vi "getConfig.vi"(6 "Delay between send and receive [ms]":i32=100, 8 "error in (no error)":errorcluster, 11 "Monochromator in":refnum<class "Monochromator.lvclass">) -> (0 "error out":errorcluster, 3 "Monochromator out":refnum<class "Monochromator.lvclass">)   [LabVIEW 2023, in "Monochromator.lvclass"]
uses:
  Monochromator.lvclass
  Monochromator.lvclass/Monochromator.ctl
  d9b87029-586e-44ee-a6e5-d4a5e0edce38.vi
  b59fd1e7-dcda-425c-bd6c-61aafb79e7f4.vi
  GenericDevice/GenericDevice.lvclass
  <vilib>/IlluminatedG/lv-web-crypto/lv-json/JSON/JSON.lvlib
panel:
  # "Connector Pane"
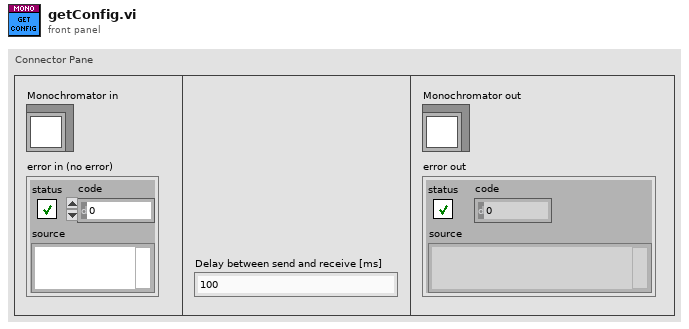
[diagram p1: front panel]
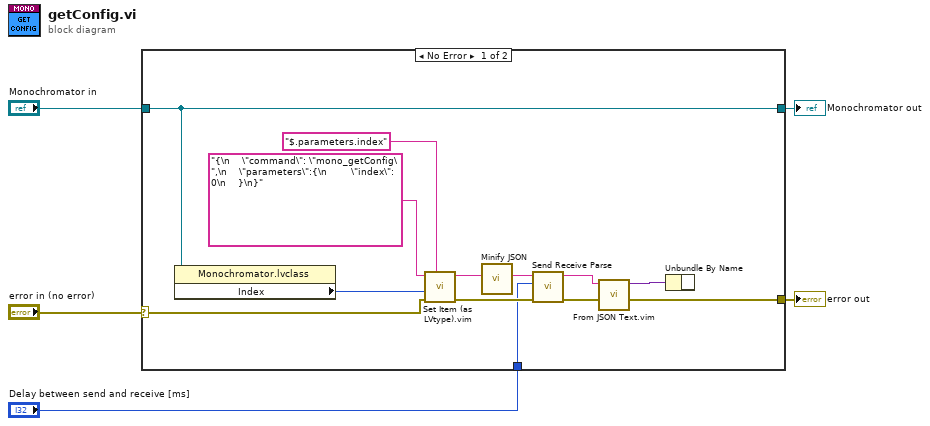
[diagram p0: block diagram]
diagram:
  n1 = case shown="No Error" "error in (no error)" {
    selector: "error in (no error)" -> [w14 w20]
    tunnel: [w13 w20] -> w4
    tunnel: [w16 w19] -> w2
    tunnel: "Monochromator in" -> [w16 w19]
    tunnel: "Delay between send and receive [ms]" -> [w6 _]
    frame No Error {
      n2 = property class="Monochromator.lvclass"(reference=w16) -> ("Index"=w15:i32)  [unwired: 1 in, 2 out]
      n3 = call "Set Item (as LVtype).vim"("$Path or Item Name"="$.parameters.index", "error in (no error)"=w14, "Anything"=w15, "JSON"="{\n    \"command\": \"mono_getConfig\",\n    \"parameters\":{\n        \"index\": 0\n    }\n}") -> ("error out"=w12:errorcluster, "<JSON>"=w9:string)  [unwired: 4 in, 1 out]
      n4 = call <vilib>:"Minify JSON.vi"("JSON String"=w9) -> ("Minified JSON"=w8:string)  [unwired: 10 in]
      n5 = call "Send Receive Parse.vi"("error in"=w12, "Delay between send and receive [ms]"=w6, "<JSON>"=w8) -> ("error out"=w10:errorcluster, "results-JSON string"=w11:string)  [unwired: 6 in, 1 out]
      n6 = call "From JSON Text.vim"("error in (no error)"=w10, "JSON"=w11) -> ("error out"=w13:errorcluster, "Data out"=w7:variant)  [unwired: 8 in]
      n7 = Unbundle By Name(w7) -> ()  [unwired: 1 out]
    }
    frame Error {
    }
  }
  "error out" <- w4
  "Monochromator out" <- w2
